vi "ATF-Pump-Seq DO Executer.vi"(8 "error in":errorcluster) -> (0 "error IO":errorcluster)   [LabVIEW 2022 SP3]
uses:
  <vilib>/Platform/TimedLoop/XDataNode/timing_clust.ctl
  <vilib>/Platform/TimedLoop/XDataNode/nitl_modes.ctl
  <vilib>/Platform/TimedLoop/XDataNode/wakeup.ctl
  05cf45a1-4425-418b-b38e-5c21057b3215.vi
  <vilib>/platform/TimedLoop/XDataNode/XDataNode.xnode
  <vilib>/Platform/TimedLoop/XDataNode/XDNodeRunTimeDep.lvlib
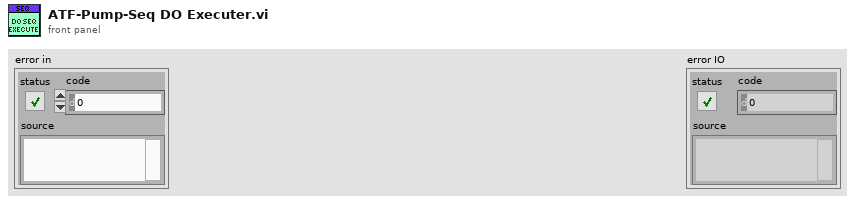
[diagram p1: front panel]
types:
  T1 = cluster{"Value":bool[], "Name":string[], "SEQ":string[], "index":i32}
  T2 = typedef "XDNodeRunTimeDep.lvlib/timing_clust.ctl" = cluster{"Expected End [f-1]":u64, "Actual End [f-1]":u64, "Finished Late? [f-1]":bool, "Expected End [i-1]":u64, "Actual End [i-1]":u64, "Finished Late? [i-1]":bool, "Expected Start [i]":u64, "Actual Start [i]":u64, "Expected Start [f]":u64, "Actual Start [f]":u64, "Source Name":string, "Structure Name":string, "Period":i64, "Deadline":i64, "Offset":i64, "Start":i64, "Priority":i32, "Timeout":i32, "Mode":T3, "Wakeup Reason":T4, "Error":errorcluster, "Source Type":string, "Secondary Source Type":string, "Global End Time":u64, "Global Start Time":u64, "Frame Duration":u64, "Iteration Duration":u64, "Assigned CPU":i32, "I/O Scan Engine Mode":u32}
  T3 = typedef "XDNodeRunTimeDep.lvlib/nitl_modes.ctl" = enum32{"No Change", "Process missed periods, maintain original phase", "Discard missed periods, maintain original phase", "Process missed periods, ignore original phase", "Discard missed periods, ignore original phase"}
  T4 = typedef "XDNodeRunTimeDep.lvlib/wakeup.ctl" = enum32{"Normal", "Aborted", "Asynchronous wakeup", "Timing source error", "Timed loop error", "Timeout"}
  T5 = enum16{"Init", "Read", "Write 'All'", "Write 'n'", "Write Safe Value", "Write Start Time", "Overwrite Pattern", "Overwrite Pattern with Start", "Append Pattern", "Start Pattern Mode", "Abort Pattern Mode", "Read 1"}
  T6 = cluster{"Start DAQ":bool, "Stop DAQ":bool, "RT Stop":bool, "RT Exit":bool, "Start Seq":bool}
  T7 = cluster{"Manual HOLD":bool, "Automatic Hold AI":bool, "Abort":bool, "Automatic Hold DI":bool}
  T8 = cluster{cluster{"Sr. No.":string, "Time CDT":string, "Component ID":string, "Data Type":string, "Condition":string, "Range/Position":string, "No of Samples for Pass":string, "Event Duration":string, "Continuous /Cumulative":string, "Expected Delay":string, "Failure case Seq":string, "Current Sequence":string}[]}[]
  T9 = cluster{cluster{"Sr. No.":string, "Time CDT":string, "Component ID":string, "Data Type":string, "Condition":string, "Range/Position":string, "No of Samples for Pass":string, "Event Duration":string, "Continuous /Cumulative":string, "Expected Delay":string, "Failure case Seq":string, "Current Sequence":string}[]}
  T10 = cluster{"Sr. No.":string, "Time CDT":string, "Component ID":string, "Data Type":string, "Condition":string, "Range/Position":string, "No of Samples for Pass":string, "Event Duration":string, "Continuous /Cumulative":string, "Expected Delay":string, "Failure case Seq":string, "Current Sequence":string}[]
  T11 = cluster{"Sr. No.":string, "Time CDT":string, "Component ID":string, "Data Type":string, "Condition":string, "Range/Position":string, "No of Samples for Pass":string, "Event Duration":string, "Continuous /Cumulative":string, "Expected Delay":string, "Failure case Seq":string, "Current Sequence":string}
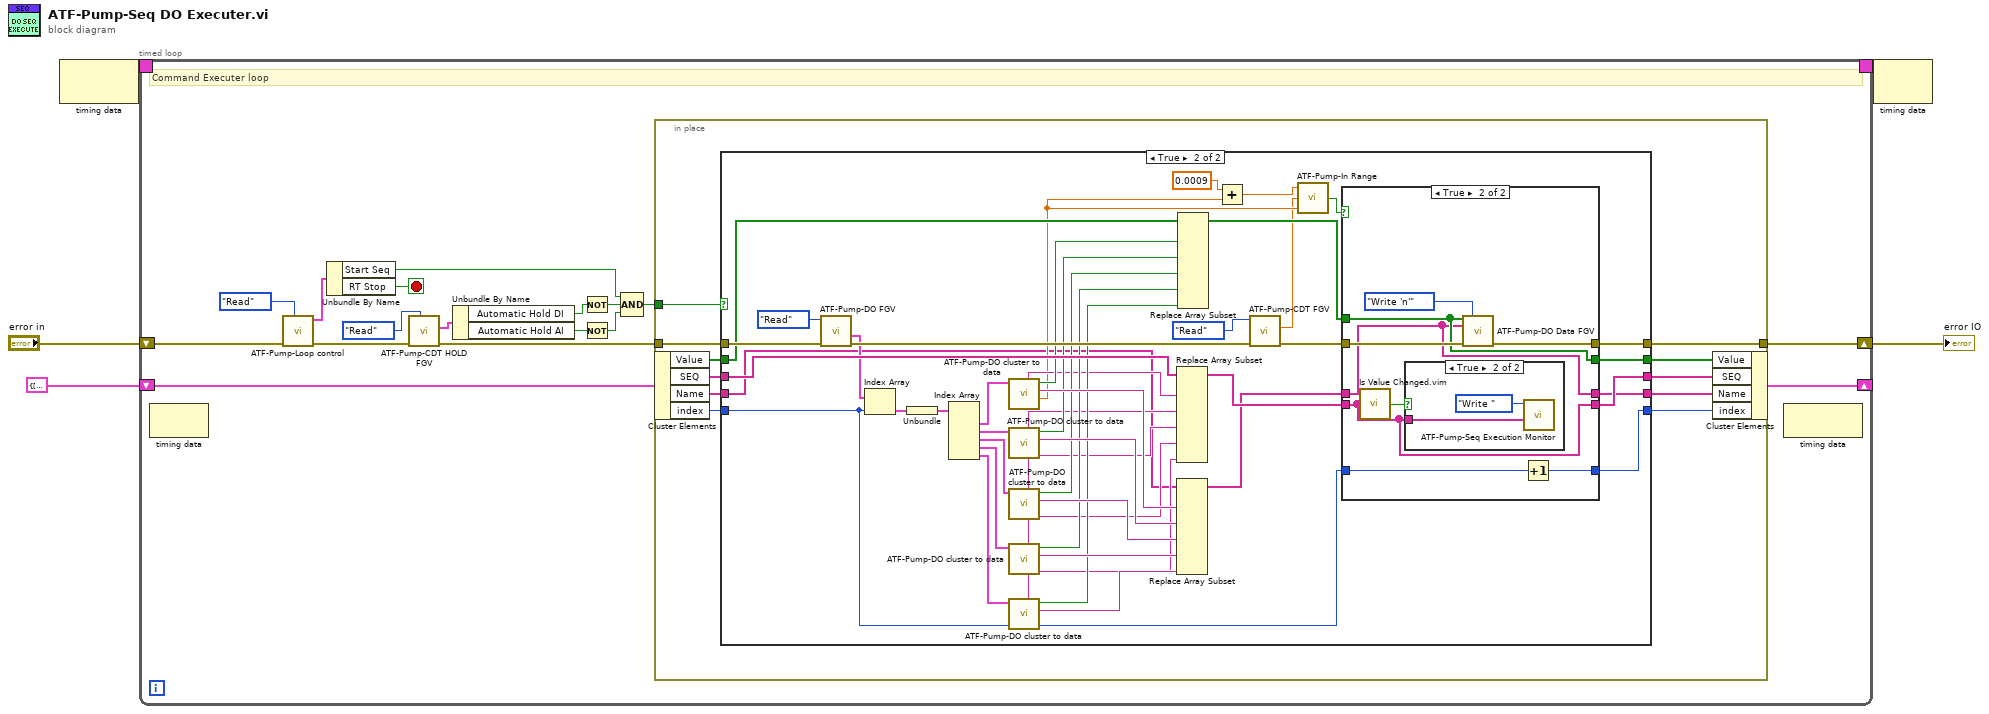
[diagram p0: block diagram]
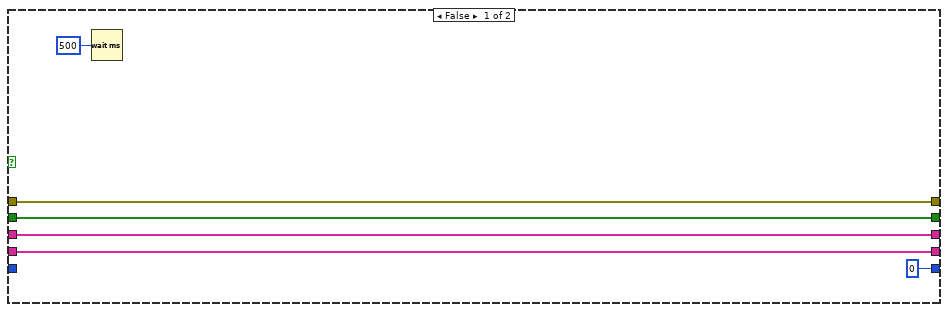
[diagram p2: hidden frame]
diagram:
  n1 = node-c288() -> (w3:T2)  [unwired: 1 in]
  n2 = timed-loop {
    shift-right: [w18] -> w4
    shift-left: "error in" -> [w21]
    timing: w3 -> [_]
    timing-out: [_] -> w2
    shift-right: [w6] -> _
    shift-left: T1 {"Value"=[FALSE, FALSE, FALSE, FALSE, FALSE], "Name"=["", "", "", "", ""], "SEQ"=["", "", "", "", ""], "index"=0} -> [w7]
    stop <- w22 stop-if-true
    # "Command Executer loop"
    n3 = node-c288() -> ()  [unwired: 1 in, 1 out]
    n4 = call "ATF-Pump-Loop control.vi"("Action"=enum16{"Init", "Write", "Read"}."Read", "error in (no error)"=w21) -> ("error Out"=w10:errorcluster, "Loop Control out"=w19:T6)  [unwired: 8 in]
    n5 = Unbundle By Name(w19) -> ("Start Seq"=w8:bool, "RT Stop"=w22:bool)
    n6 = call "ATF-Pump-CDT HOLD FGV.vi"("Write/Read"=enum16{"Write", "Read"}."Read", "error in (no error)"=w10) -> ("error Out"=w9:errorcluster, "HOLD and Abort Out"=w14:T7)  [unwired: 6 in]
    n7 = Unbundle By Name(w14) -> ("Automatic Hold DI"=w12:bool, "Automatic Hold AI"=w13:bool)
    n8 = Not(x=w12) -> (.not. x?=w11:bool)
    n9 = Not(x=w13) -> (.not. x?=w16:bool)
    n10 = Compound Arithmetic op=AND(w8, w11, w16) -> (w15:bool)
    n11 = in-place "In Place Element Structure" {
      in-place-border: [w33] -> w18
      in-place-border: w15 -> [w32]
      in-place-border: w9 -> [w31]
      n12 = in-place-cluster #1(w7) -> ("Value"=w30:bool[], "SEQ"=w29:string[], "Name"=w28:string[], "index"=w27:i32)
      n13 = case shown="True" w32 {
        tunnel: w31 -> [w39 w83]
        tunnel: [w39 w81] -> w33
        tunnel: w29 -> [w35 w80]
        tunnel: w30 -> [w37 w79]
        tunnel: [w37 w43] -> w23
        tunnel: [w34 w40] -> w25
        tunnel: [w35 w41] -> w26
        tunnel: w27 -> [_ w44]
        tunnel: [0 ("index") w45] -> w24
        tunnel: w28 -> [w34 w42]
        frame False {
          n14 = Wait (ms)(milliseconds to wait=u32 500) -> ()  [unwired: 1 out]
        }
        frame True {
          n15 = call "ATF-Pump-DO FGV.vi"("error in"=w83, "Enum"=enum16{"Read", "Write "}."Read") -> ("error out"=w82:errorcluster, "DO Seq  OUT"=w76:T8)  [unwired: 8 in]
          n16 = Index Array(array=w76, index=w44) -> (element=w75:T9)
          n17 = Unbundle(w75) -> (w74:T10)
          n18 = Index Array(array=w74) -> (element #1=w51:T11, element #2=w73:T11, element #3=w72:T11, element #4=w71:T11, element #5=w70:T11)  [unwired: 5 in]
          n19 = call "ATF-Pump-DO cluster to data.vi"("output cluster"=w51) -> ("Numeric"=w49:dbl, "Component ID"=w68:string, "Boolean"=w63:bool, "Sequence"=w56:string)  [unwired: 7 in]
          n20 = call "ATF-Pump-DO cluster to data.vi"("output cluster"=w73) -> ("Component ID"=w67:string, "Boolean"=w62:bool, "Sequence"=w55:string)  [unwired: 7 in, 1 out]
          n21 = call "ATF-Pump-DO cluster to data.vi"("output cluster"=w72) -> ("Component ID"=w66:string, "Boolean"=w61:bool, "Sequence"=w54:string)  [unwired: 7 in, 1 out]
          n22 = call "ATF-Pump-DO cluster to data.vi"("output cluster"=w71) -> ("Component ID"=w65:string, "Boolean"=w60:bool, "Sequence"=w53:string)  [unwired: 7 in, 1 out]
          n23 = call "ATF-Pump-DO cluster to data.vi"("output cluster"=w70) -> ("Component ID"=w64:string, "Boolean"=w59:bool, "Sequence"=w52:string)  [unwired: 7 in, 1 out]
          n24 = Replace Array Subset(array=w80, new element #1=w56, new element #2=w55, new element #3=w54, new element #4=w53, new element #5=w52) -> (w78:string[])  [unwired: 5 in]
          n25 = Replace Array Subset(array=w42, new element #1=w68, new element #2=w67, new element #3=w66, new element #4=w65, new element #5=w64) -> (w77:string[])  [unwired: 5 in]
          n26 = Replace Array Subset(array=w79, new element #1=w63, new element #2=w62, new element #3=w61, new element #4=w60, new element #5=w59) -> (w58:bool[])  [unwired: 5 in]
          n27 = Add(x=0.0009, y=w49) -> (x+y=w50:dbl)
          n28 = call "ATF-Pump-CDT FGV.vi"("error in (no error)"=w82, "Write/Read"=enum16{"Write", "Read"}."Read") -> ("error Out"=w57:errorcluster, "CDT Out"=w47:dbl)  [unwired: 8 in]
          n29 = call "ATF-Pump-In Range.vi"("Min"=w49, "X"=w47, "Max"=w50) -> ("In Range"=w46:bool)  [unwired: 2 in]
          n30 = case shown="True" w46 {
            tunnel: w57 -> [w89 w98]
            tunnel: [w89 w97] -> w81
            tunnel: w58 -> [w88 w94]
            tunnel: w77 -> [w85 w90]
            tunnel: w78 -> [w86 w91]
            tunnel: [w88 w94] -> w43
            tunnel: [w87 w92] -> w45
            tunnel: w44 -> [w87 w93]
            tunnel: [w86 w91] -> w41
            tunnel: [w85 w90] -> w40
            frame False {
            }
            frame True {
              n31 = call "Is Value Changed.vim"("value"=w91) -> ("changed or first call?"=w95:bool)
              n32 = case shown="True" w95 {
                tunnel: w91 -> [_ w100]
                frame False {
                }
                frame True {
                  n33 = call "ATF-Pump-Seq Execution Monitor.vi"("Seq Monitor"=w100, "Enum"=enum16{"Read", "Write "}."Write ") -> ()  [unwired: 8 in, 2 out]
                }
              }
              n34 = call "ATF-Pump-DO Data FGV.vi"("DO Values In"=w94, "Option"=T5."Write 'n'", "DO Channel Names"=w90, "error in (no error)"=w98) -> ("error out"=w97:errorcluster)  [unwired: 5 in, 6 out]
              n35 = Increment(x=w93) -> (x+1=w92:i32)
            }
          }
        }
      }
      n36 = in-place-cluster #1("Value"=w23, "SEQ"=w26, "Name"=w25, "index"=w24) -> (w6:T1)
    }
    n37 = node-c288() -> ()  [unwired: 1 in, 1 out]
  }
  "error IO" <- w4
  n38 = node-c288(w2) -> ()  [unwired: 1 out]
